vi "Save datapoint2.vi"(8 "error in (no error)":errorcluster, 9 "Data in":T2, 10 "Instruments":T1 {"SMU 2"."Last updated" format="%<%H:%M:%S>T"; "SMU 1"."Last updated" format="%<%H:%M:%S>T"; "TC"."Last updated" format="%<%H:%M:%S>T"}, 11 "graph data in":cluster{"Array":dbl[], "Array":dbl[]}[](array[cluster])) -> (0 "error out":errorcluster, 1 "Is complete":bool, 2 "Data out":T2, 3 "Progress %":dbl(slide) caption="Horizontal Pointer Slide" scale=0.0..100.0, 5 "Graph data out":cluster{"Array":dbl[], "Array":dbl[]}[](array[cluster]))   [LabVIEW 2021]
doc: "Writes datapoint in TDMS file"
uses:
  controls/Data.ctl
  <vilib>/GPower/Math/Library/Percent/PercentT/PTI32.vi
  <vilib>/GPower/Math/GPMath.lvlib
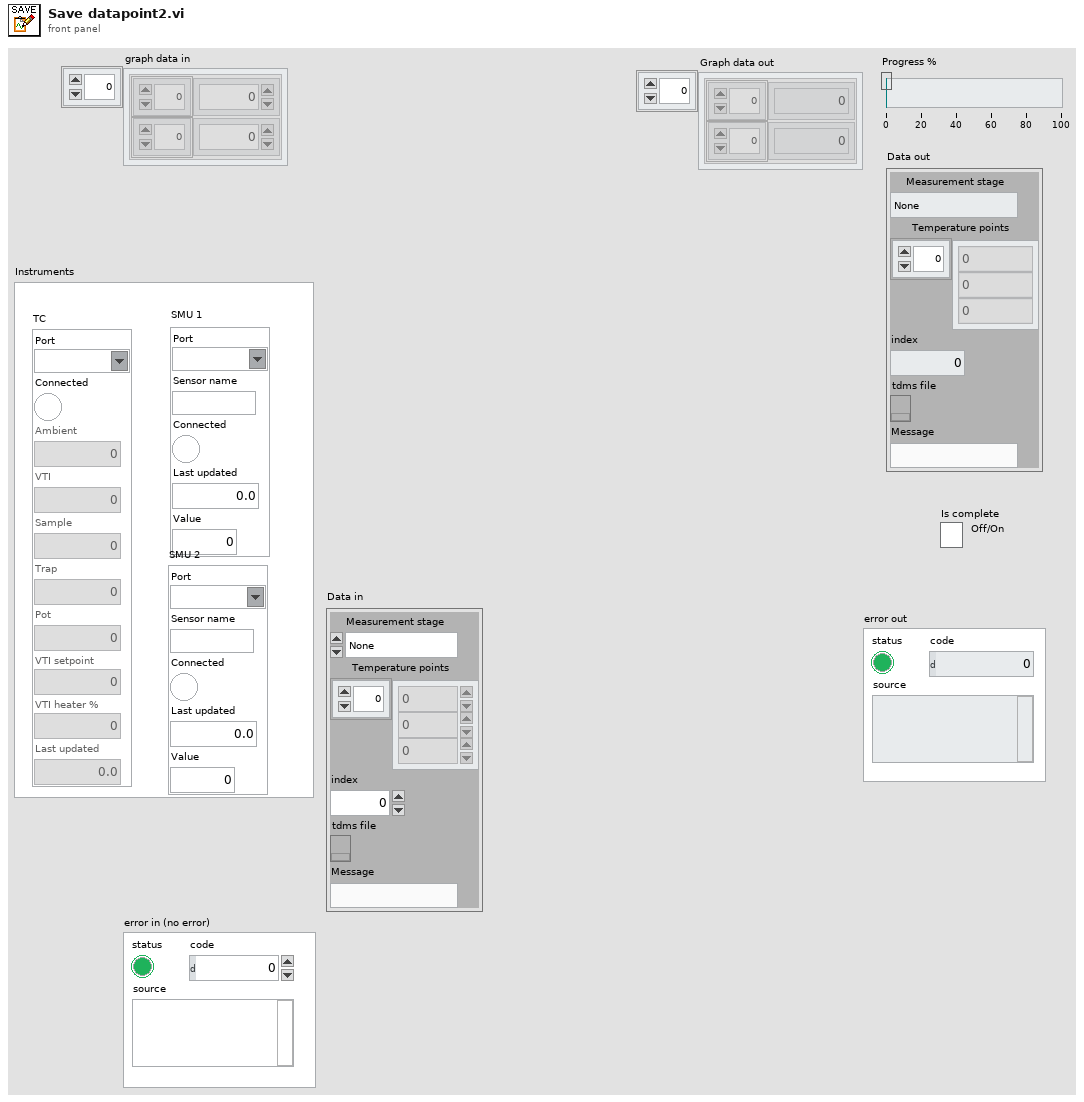
[diagram p1: front panel]
types:
  T1 = cluster{"TC":cluster{"Port":refnum<visa-resource-name>, "Connected":bool, "Ambient":dbl, "VTI":dbl, "Sample":dbl, "Trap":dbl, "Pot":dbl, "VTI setpoint":dbl, "VTI heater %":dbl, "Last updated":dbl}, "SMU 1":cluster{"Port":refnum<visa-resource-name>, "Sensor name":string, "Connected":bool, "Last updated":dbl, "Value":dbl}, "SMU 2":cluster{"Port":refnum<visa-resource-name>, "Sensor name":string, "Connected":bool, "Last updated":dbl, "Value":dbl}}
  T2 = typedef "Data.ctl" = cluster{"Measurement stage":enum16{"None", "Wait to start", "Stage 1", "Interstage", "Stage 2", "Stopping"}, "Temperature points":dbl[], "index":i32, "tdms file":refnum<k34>, "Message":string}
  T3 = enum16{"None", "Wait to start", "Stage 1", "Interstage", "Stage 2", "Stopping"}
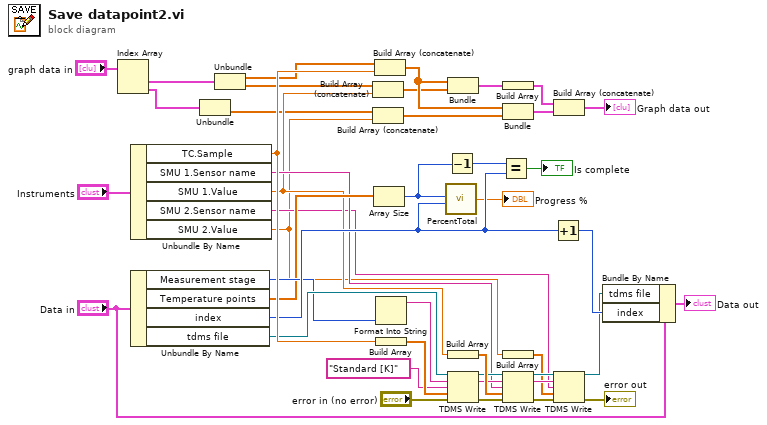
[diagram p0: block diagram]
diagram:
  n1 = Index Array(array="graph data in") -> (element #1=w38:cluster{"Array":dbl[], "Array":dbl[]}, element #2=w44:cluster{"Array":dbl[], "Array":dbl[]})  [unwired: 2 in]
  n2 = Unbundle By Name("Instruments") -> ("TC.Sample"=w42:dbl, "SMU 1.Sensor name"=w8:string, "SMU 1.Value"=w7:dbl, "SMU 2.Sensor name"=w5:string, "SMU 2.Value"=w3:dbl)
  n3 = Unbundle By Name("Data in") -> ("Measurement stage"=w19:T3, "Temperature points"=w15:dbl[], "index"=w30:i32, "tdms file"=w20:refnum<k34>)
  n4 = Unbundle(w44) -> ("Array"=w4:dbl[])  [unwired: 1 out]
  n5 = Unbundle(w38) -> ("Array"=w39:dbl[], "Array"=w40:dbl[])
  n6 = Build Array (concatenate)(w40, w7) -> (w41:dbl[])
  n7 = Build Array (concatenate)(w4, w3) -> (w1:dbl[])
  n8 = Array Size(array=w15) -> (size(s)=w12:i32)
  n9 = Build Array (concatenate)(w39, w42) -> (w43:dbl[])
  n10 = Format Into String(w19) -> (resulting string=w18:string)  [unwired: 3 in, 1 out]
  n11 = Build Array(w42) -> (w35:dbl[])
  n12 = call-poly <vilib>:"PercentTotal.vi"("b"=w30, "a"=w12) -> ("b % total of a"=→"Progress %":dbl)  [unwired: 4 in]
  n13 = Decrement(x=w12) -> (x-1=w11:i32)
  n14 = Bundle(w43, w41) -> (w32:cluster{dbl[], dbl[]})  [unwired: 1 in]
  n15 = Build Array(w7) -> (w34:dbl[])
  n16 = TDMS Write(0:w20, 5:w18, 7:"Standard [K]", 9:w35, 11:"error in (no error)") -> (4:w16:refnum<k34>, 6:w22:string, 15:w17:errorcluster)  [unwired: 1 in, 1 out]
  n17 = Equal?(x=w11, y=w30) -> (x = y?=→"Is complete":bool)
  n18 = Build Array(w32) -> (w33:cluster{dbl[], dbl[]}[])
  n19 = Bundle(w43, w1) -> (w6:cluster{dbl[], dbl[]})  [unwired: 1 in]
  n20 = Build Array(w3) -> (w2:dbl[])
  n21 = TDMS Write(0:w16, 5:w22, 7:w8, 9:w34, 11:w17) -> (4:w23:refnum<k34>, 6:w24:string, 15:w25:errorcluster)  [unwired: 1 in, 1 out]
  n22 = Increment(x=w30) -> (x+1=w31:i32)
  n23 = Build Array (concatenate)(w33, w6) -> (→"Graph data out":cluster{dbl[], dbl[]}[])
  n24 = TDMS Write(0:w23, 5:w24, 7:w5, 9:w2, 11:w25) -> (4:w29:refnum<k34>, 15:→"error out":errorcluster)  [unwired: 1 in, 2 out]
  n25 = Bundle By Name(cluster="Data in", "tdms file"=w29, "index"=w31) -> (→"Data out":T2)
